vi "Write_data_file.vi"(2 "error in":errorcluster, 3 "Latest_Data":T1 {"Temperature" scale=0.0..100.0; "Pressure (barg)" scale=0.0..70.0}, 4 "Input file refnum":refnum<file>) -> (0 "error out":errorcluster, 1 "output file refnum":refnum<file>)   [LabVIEW 2016]
uses:
  adsorbed_cluster.ctl
panel:
  in  "VISA resource name":refnum<visa-resource-name>
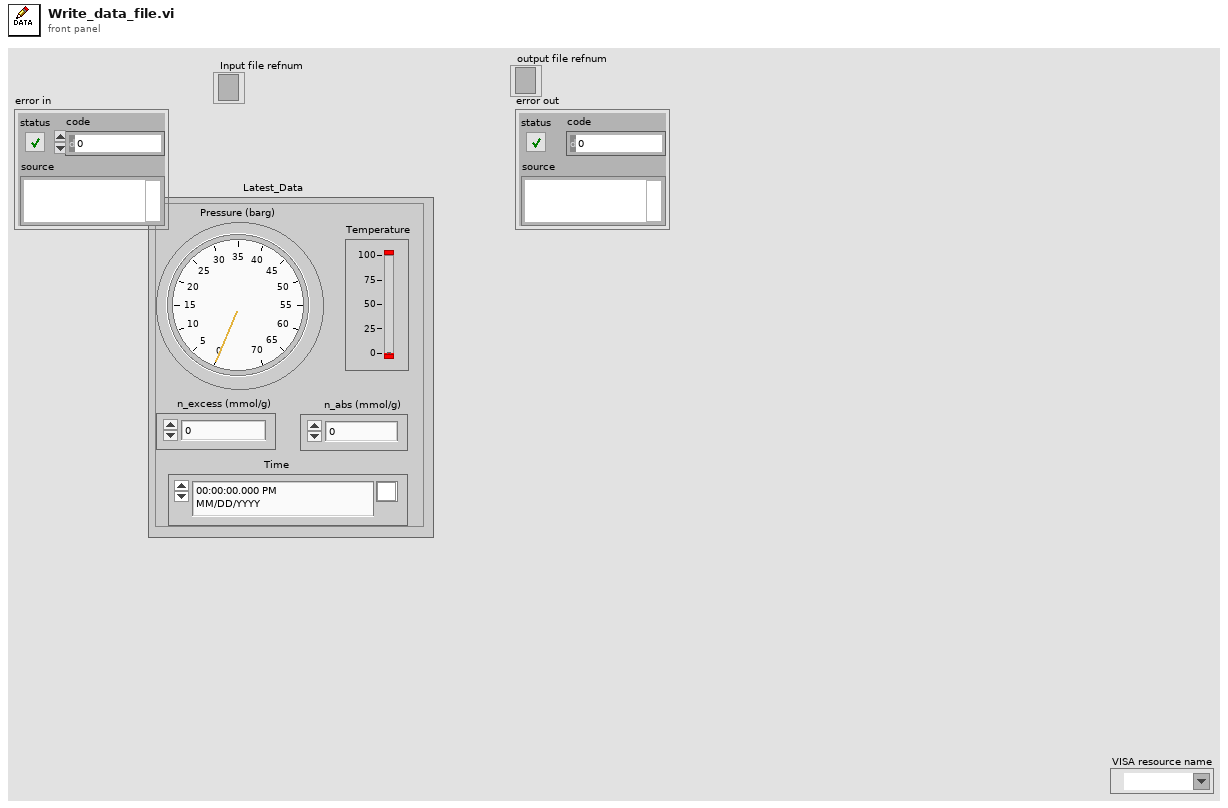
[diagram p1: front panel]
types:
  T1 = typedef "adsorbed_cluster.ctl" = cluster{"Time":timestamp, "Pressure (barg)":dbl, "n_excess (mmol/g)":dbl, "n_abs (mmol/g)":dbl, "Temperature":dbl}
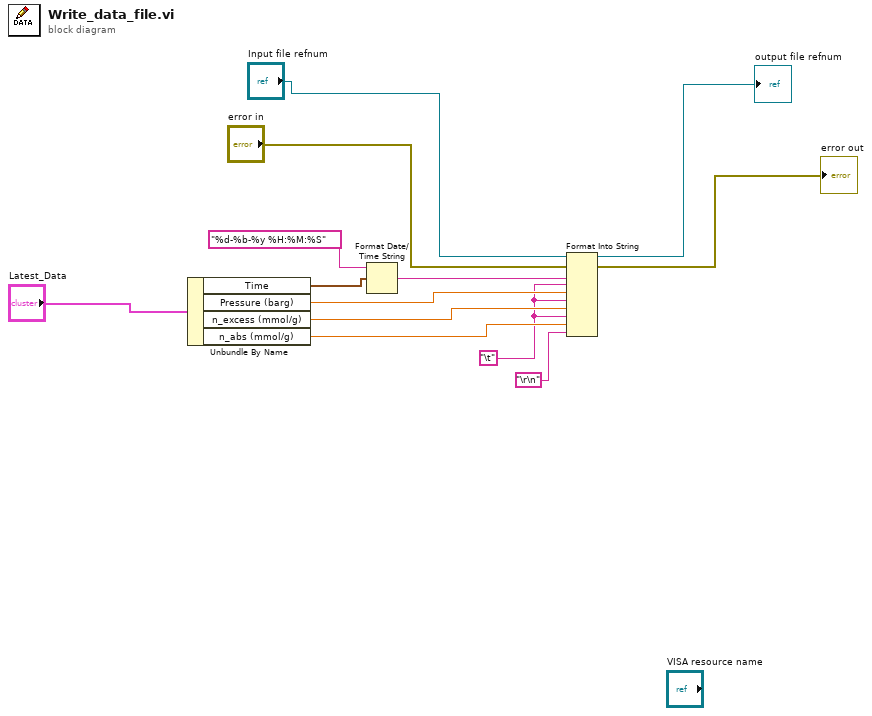
[diagram p0: block diagram]
diagram:
  w5 = "\t"
  n1 = Unbundle By Name("Latest_Data") -> ("Time"=w12:timestamp, "Pressure (barg)"=w8:dbl, "n_excess (mmol/g)"=w7:dbl, "n_abs (mmol/g)"=w6:dbl)
  n2 = Format Date/Time String(time format string (%c)="%d-%b-%y %H:%M:%S", seconds (now)=w12) -> (date/time string=w10:string)  [unwired: 1 in]
  n3 = Format Into String(initial string="Input file refnum", error in="error in", w10, w5, w8, w5, w7, w5, w6, "\r\n") -> (resulting string=→"output file refnum":refnum<file>, error out=→"error out":errorcluster)  [unwired: 1 in]
